vi "Get Master and Slave Tasks.vi"(8 "error in (no error)":errorcluster, 10 "AI tasks in":refnum<k21>[](array[refnum]), 11 "AI task":refnum<k21>) -> (0 "error out":errorcluster, 2 "master task":refnum<k21>, 3 "AI task out":refnum<k21>)   [LabVIEW 2019, in "Instrument.DAQ.lvclass"]
uses:
  Instrument.DAQ.lvclass
  <userlib>/_OpenG.lib/array/array.llb/Search 1D Array (U32)__ogtk.vi
  <userlib>/_OpenG.lib/array/array.llb/Index 1D Array Elements (U32)__ogtk.vi
  <resource>/objmgr/daqmx.rc
panel:
  out "x-y":dbl
  out "Slots":u32[](array[numeric])
  out "Chassis":u32[](array[numeric])
  out "Devices":tag[](array[tag])
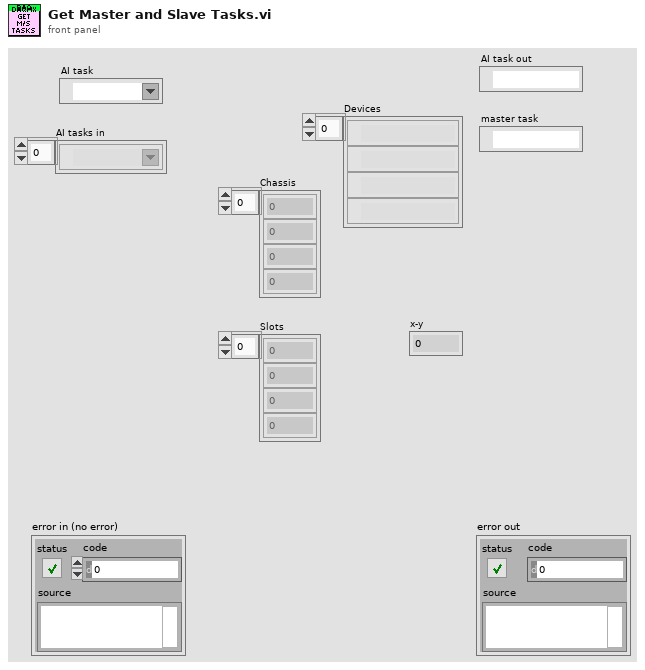
[diagram p1: front panel]
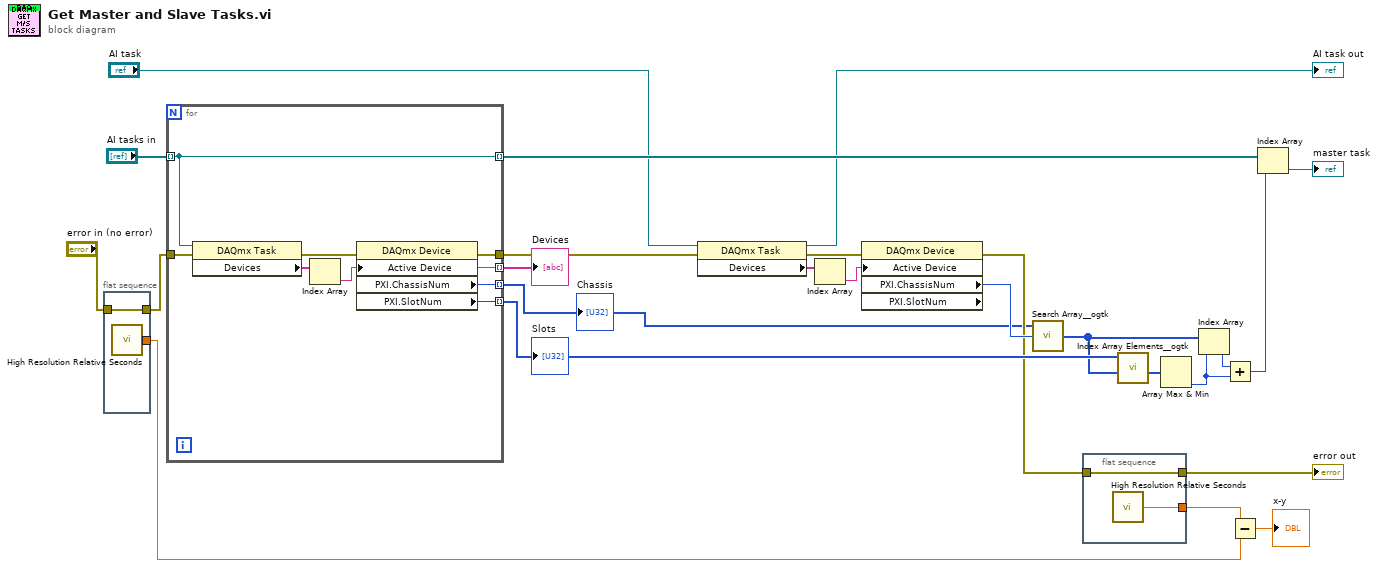
[diagram p0: block diagram]
diagram:
  n1 = flat-sequence {
    tunnel: [w27] -> w14
    tunnel: "error in (no error)" -> [w27]
    tunnel: [w26] -> w9
    frame #0 {
      n2 = call <vilib>:"High Resolution Relative Seconds.vi"() -> ("relative seconds"=w26:dbl)
    }
  }
  n3 = for {
    tunnel: "AI tasks in" -> [w30] mode=indexing
    tunnel: [w30] -> w15 mode=indexing
    tunnel: [w33] -> w1 mode=indexing
    tunnel: [w31] -> w24 mode=indexing
    tunnel: [w32] -> w18 mode=indexing
    tunnel: [w29] -> w20
    tunnel: w14 -> [w28]
    n4 = property class="DAQmx Task"(reference=w30, error in=w28) -> (error out=w35:errorcluster, "Devices"=w34:tag[])  [unwired: 1 out]
    n5 = Index Array(array=w34) -> (element=w31:tag)  [unwired: 1 in]
    n6 = property class="DAQmx Device"(error in=w35, "Active Device"=w31) -> (error out=w29:errorcluster, "PXI.ChassisNum"=w33:u32, "PXI.SlotNum"=w32:u32)  [unwired: 1 in, 1 out]
  }
  "Devices" <- w24
  "Chassis" <- w1
  "Slots" <- w18
  n7 = property class="DAQmx Task"(reference="AI task", error in=w20) -> (reference out=→"AI task out":refnum<k21>, error out=w21:errorcluster, "Devices"=w22:tag[])
  n8 = Index Array(array=w22) -> (element=w23:tag)  [unwired: 1 in]
  n9 = property class="DAQmx Device" props=["Active Device", "PXI.ChassisNum", "PXI.SlotNum"](error in=w21, "Active Device"=w23) -> (error out=w11:errorcluster, "PXI.ChassisNum"=w19:u32)  [unwired: 1 in, 2 out]
  n10 = call-poly <userlib>:"Search Array__ogtk.vi"("Array"=w1, "Element Data"=w19) -> ("Indices of Elements"=w7:i32[])  [unwired: 7 in]
  n11 = flat-sequence {
    tunnel: [w37] -> w12
    tunnel: w11 -> [w37]
    tunnel: [w36] -> w10
    frame #0 {
      n12 = call <vilib>:"High Resolution Relative Seconds.vi"() -> ("relative seconds"=w36:dbl)
    }
  }
  n13 = call-poly <userlib>:"Index Array Elements__ogtk.vi"("indices"=w7, "array"=w18) -> ("elements"=w17:u32[])  [unwired: 9 in]
  n14 = Array Max & Min(array=w17) -> (min index (indices)=w6:i32)  [unwired: 3 out]
  n15 = Index Array(array=w7, index=w6) -> (element=w5:i32)
  n16 = Add(x=w5, y=w6) -> (x+y=w2:i32)
  n17 = Subtract(x=w10, y=w9) -> (x-y=→"x-y":dbl)
  n18 = Index Array(array=w15, index=w2) -> (element=→"master task":refnum<k21>)
  "error out" <- w12
